vi "myDLTS GUID.vi"(1 "Method":T1(ring)) -> (0 "GUID":string)   [LabVIEW 2019]
doc: "Generates GUID using various methods"
uses:
  <vilib>/numeric/Random Number (Range) U64.vi
  <vilib>/numeric/sub_Random U32.vi
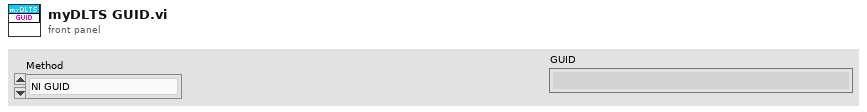
[diagram p1: front panel]
types:
  T1 = enum16{"NI GUID", "Windows GUID", "Random GUID 4", "Return"}
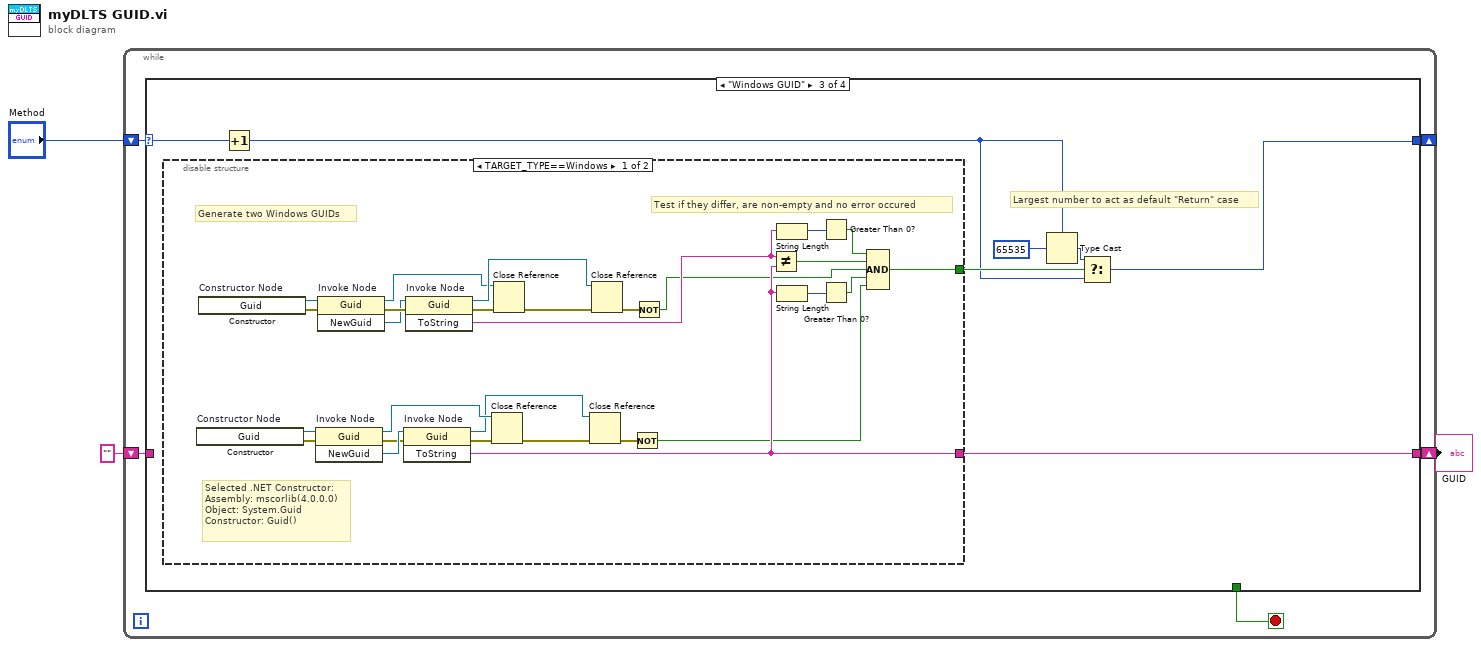
[diagram p0: block diagram]
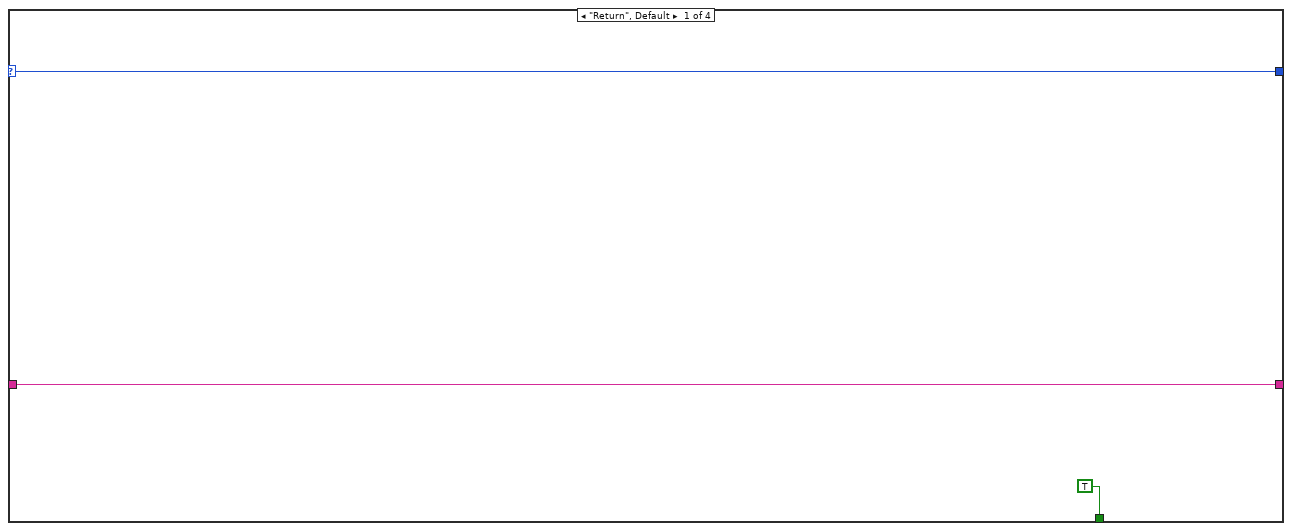
[diagram p2: hidden frame]
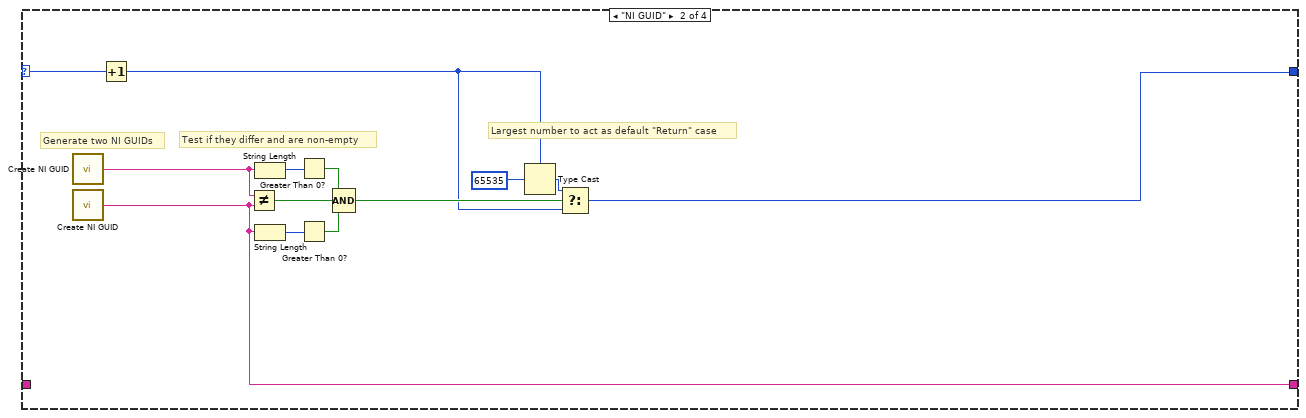
[diagram p3: hidden frame]
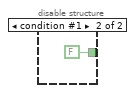
[diagram p4: hidden frame]
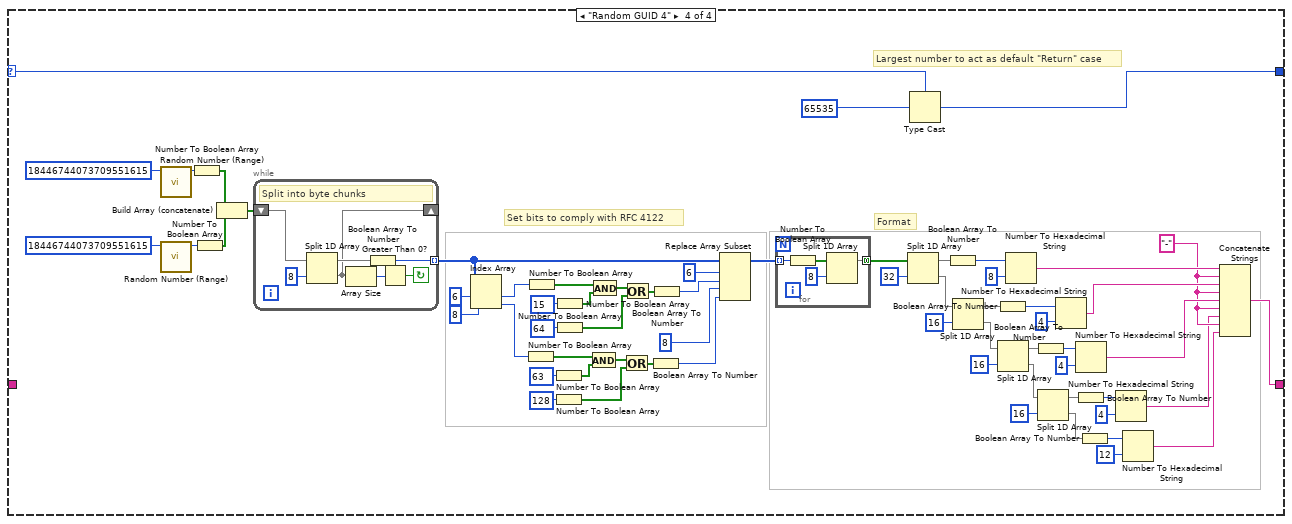
[diagram p5: hidden frame]
diagram:
  n1 = while {
    shift-right: [w7] -> _
    shift-left: "Method" -> [w8]
    shift-right: [w5] -> w1
    shift-left: "" ("NI GUID") -> [w4]
    stop <- w6 stop-if-true
    n2 = case shown="\"Windows GUID\"" w8 {
      selector: w8 -> [w9 w17 w30 w124]
      tunnel: [w9 w16 w29 w122] -> w7
      tunnel: [TRUE _ _ _] -> w6
      tunnel: [w10 w15 w25 w62] -> w5
      tunnel: w4 -> [w10 _ _ _]
      frame "Return", Default {
      }
      frame "NI GUID" {
        # "Largest number to act as default \"Return\" case"
        # "Test if they differ and are non-empty"
        # "Generate two NI GUIDs"
        n3 = call "Create NI GUID.vi"() -> ("NI GUID"=w24:string)
        n4 = call "Create NI GUID.vi"() -> ("NI GUID"=w15:string)
        n5 = Increment(x=w17) -> (x+1=w14:T1)
        n6 = Not Equal?(x=w24, y=w15) -> (x != y?=w20:bool)
        n7 = String Length(string=w24) -> (length=w23:i32)
        n8 = String Length(string=w15) -> (length=w22:i32)
        n9 = Greater Than 0?(x=w23) -> (x > 0?=w21:bool)
        n10 = Greater Than 0?(x=w22) -> (x > 0?=w19:bool)
        n11 = Compound Arithmetic op=AND(w21, w20, w19) -> (w18:bool)
        n12 = Type Cast(type=w14, x=u16 65535) -> (*(type *) &x=w12:T1)
        n13 = Select(t=w12, s=w18, f=w14) -> (s? t:f=w16:T1)
      }
      frame "Windows GUID" {
        # "Largest number to act as default \"Return\" case"
        n14 = disable-structure shown="TARGET_TYPE==Windows" {
          disable-tunnel: [w55 FALSE] -> w31
          disable-tunnel: [w37 _] -> w25
          frame condition #0 (active) {
            # "Selected .NET Constructor:\nAssembly: mscorlib(4.0.0.0)\nObject: System.Guid\nConstructor: Guid()"
            # "Test if they differ, are non-empty and no error occured"
            # "Generate two Windows GUIDs"
            n15 = constructor on="Constructor Node" class="System.Guid"() -> (reference out=w54:refnum<k24>, error out=w53:errorcluster)  [unwired: 3 in, 1 out]
            n16 = constructor on="Constructor Node" class="System.Guid"() -> (reference out=w39:refnum<k24>, error out=w40:errorcluster)  [unwired: 3 in, 1 out]
            n17 = invoke on="Invoke Node" class="Guid" method="NewGuid"(reference=w54, error in=w53) -> (reference out=w48:refnum<k24>, error out=w51:errorcluster, "NewGuid"=w52:refnum<k24>)  [unwired: 1 in]
            n18 = invoke on="Invoke Node" class="Guid" method="NewGuid"(reference=w39, error in=w40) -> (reference out=w45:refnum<k24>, error out=w42:errorcluster, "NewGuid"=w41:refnum<k24>)  [unwired: 1 in]
            n19 = invoke on="Invoke Node" class="Guid" method="ToString"(reference=w52, error in=w51) -> (reference out=w47:refnum<k24>, error out=w50:errorcluster, "ToString"=w37:string)  [unwired: 1 in]
            n20 = invoke on="Invoke Node" class="Guid" method="ToString"(reference=w41, error in=w42) -> (reference out=w46:refnum<k24>, error out=w43:errorcluster, "ToString"=w38:string)  [unwired: 1 in]
            n21 = Close Reference(reference=w48, error in (no error)=w50) -> (error out=w49:errorcluster)
            n22 = Close Reference(reference=w45, error in (no error)=w43) -> (error out=w44:errorcluster)
            n23 = Close Reference(reference=w47, error in (no error)=w49) -> (error out=w35:errorcluster)
            n24 = Close Reference(reference=w46, error in (no error)=w44) -> (error out=w36:errorcluster)
            n25 = Not(x=w35) -> (.not. x?=w34:bool)
            n26 = Not(x=w36) -> (.not. x?=w32:bool)
            n27 = Not Equal?(x=w38, y=w37) -> (x != y?=w56:bool)
            n28 = String Length(string=w38) -> (length=w59:i32)
            n29 = String Length(string=w37) -> (length=w58:i32)
            n30 = Greater Than 0?(x=w59) -> (x > 0?=w57:bool)
            n31 = Greater Than 0?(x=w58) -> (x > 0?=w33:bool)
            n32 = Compound Arithmetic op=AND(w57, w56, w32, w33, w34) -> (w55:bool)
          }
          frame condition #1 {
          }
        }
        n33 = Increment(x=w30) -> (x+1=w28:T1)
        n34 = Type Cast(type=w28, x=u16 65535) -> (*(type *) &x=w26:T1)
        n35 = Select(t=w26, s=w31, f=w28) -> (s? t:f=w29:T1)
      }
      frame "Random GUID 4" {
        w65 = "-" ("string")
        # "Format"
        # "Set bits to comply with RFC 4122"
        # "Largest number to act as default \"Return\" case"
        n36 = call-poly <vilib>:"Random Number (Range).vi"("upper bound (100)"=u64 18446744073709551615) -> ("number"=w119:u64)  [unwired: 10 in]
        n37 = call-poly <vilib>:"Random Number (Range).vi"("upper bound (100)"=u64 18446744073709551615) -> ("number"=w118:u64)  [unwired: 10 in]
        n38 = Number To Boolean Array(number=w119) -> (Boolean array=w117:bool[])
        n39 = Number To Boolean Array(number=w118) -> (Boolean array=w116:bool[])
        n40 = Build Array (concatenate)(w117, w116) -> (w93:bool[])
        n41 = while {
          tunnel: [w129] -> w61 mode=indexing
          shift-right: [w130] -> _
          shift-left: w93 -> [w134]
          stop <- w132 continue-if-true
          # "Split into byte chunks"
          n42 = Split 1D Array(array=w134, index=8) -> (first subarray=w131:bool[], second subarray=w130:bool[])
          n43 = Array Size(array=w130) -> (size(s)=w133:i32)
          n44 = Boolean Array To Number(Boolean array=w131) -> (number=w129:u32)
          n45 = Greater Than 0?(x=w133) -> (x > 0?=w132:bool)
        }
        n46 = Index Array(array=w61, index #1=6 ("index"), index #2=8 ("index")) -> (element #1=w113:u32, element #2=w97:u32)
        n47 = Number To Boolean Array(number=w97) -> (Boolean array=w104:bool[])
        n48 = Number To Boolean Array(number=w113) -> (Boolean array=w112:bool[])
        n49 = Number To Boolean Array(number=u32 63) -> (Boolean array=w103:bool[])
        n50 = Number To Boolean Array(number=u32 128) -> (Boolean array=w99:bool[])
        n51 = Number To Boolean Array(number=u32 15) -> (Boolean array=w111:bool[])
        n52 = Number To Boolean Array(number=u32 64) -> (Boolean array=w107:bool[])
        n53 = And(x=w104, y=w103) -> (x .and. y?=w101:bool[])
        n54 = And(x=w112, y=w111) -> (x .and. y?=w109:bool[])
        n55 = Or(x=w101, y=w99) -> (x .or. y?=w98:bool[])
        n56 = Or(x=w109, y=w107) -> (x .or. y?=w106:bool[])
        n57 = Boolean Array To Number(Boolean array=w98) -> (number=w95:u32)
        n58 = Boolean Array To Number(Boolean array=w106) -> (number=w96:u32)
        n59 = Replace Array Subset(array=w61, new element #1=w96, index #1=6 ("index"), new element #2=w95, index #2=8 ("index")) -> (w89:u32[])
        n60 = for {
          tunnel: w89 -> [w128] mode=indexing
          tunnel: [w126] -> w88 mode=concatenating
          n61 = Number To Boolean Array(number=w128) -> (Boolean array=w127:bool[])
          n62 = Split 1D Array(array=w127, index=8) -> (first subarray=w126:bool[])  [unwired: 1 out]
        }
        n63 = Split 1D Array(array=w88, index=32) -> (first subarray=w87:bool[], second subarray=w85:bool[])
        n64 = Type Cast(type=w124, x=u16 65535) -> (*(type *) &x=w122:T1)
        n65 = Boolean Array To Number(Boolean array=w87) -> (number=w91:u32)
        n66 = Split 1D Array(array=w85, index=16) -> (first subarray=w82:bool[], second subarray=w84:bool[])
        n67 = Boolean Array To Number(Boolean array=w82) -> (number=w79:u32)
        n68 = Split 1D Array(array=w84, index=16) -> (first subarray=w81:bool[], second subarray=w70:bool[])
        n69 = Number To Hexadecimal String(1:i16 8 ("width (-)"), 2:w91) -> (0:w68:string)
        n70 = Boolean Array To Number(Boolean array=w81) -> (number=w77:u32)
        n71 = Split 1D Array(array=w70, index=16) -> (first subarray=w73:bool[], second subarray=w69:bool[])
        n72 = Number To Hexadecimal String(1:i16 4 ("width (-)"), 2:w79) -> (0:w67:string)
        n73 = Number To Hexadecimal String(1:i16 4 ("width (-)"), 2:w77) -> (0:w66:string)
        n74 = Boolean Array To Number(Boolean array=w73) -> (number=w71:u32)
        n75 = Boolean Array To Number(Boolean array=w69) -> (number=w75:u32)
        n76 = Number To Hexadecimal String(1:i16 4 ("width (-)"), 2:w71) -> (0:w63:string)
        n77 = Number To Hexadecimal String(1:i16 12 ("width (-)"), 2:w75) -> (0:w64:string)
        n78 = Concatenate Strings(w68, w65, w67, w65, w66, w65, w63, w65, w64) -> (w62:string)
      }
    }
  }
  "GUID" <- w1
